vi "CASE.vi"() -> ()   [LabVIEW 2020]
panel:
  out "WARNING":string
  out "Boolean 5":bool
  in  "error out":errorcluster
  out "decimal integer string":string
  in  "Knob":u8(knob) scale=0.0..10.0
  in  "String 2":string
  out "Boolean 4":bool
  out "Boolean 3":bool
  out "Boolean 2":bool
  out "String":string
  in  "Boolean":bool
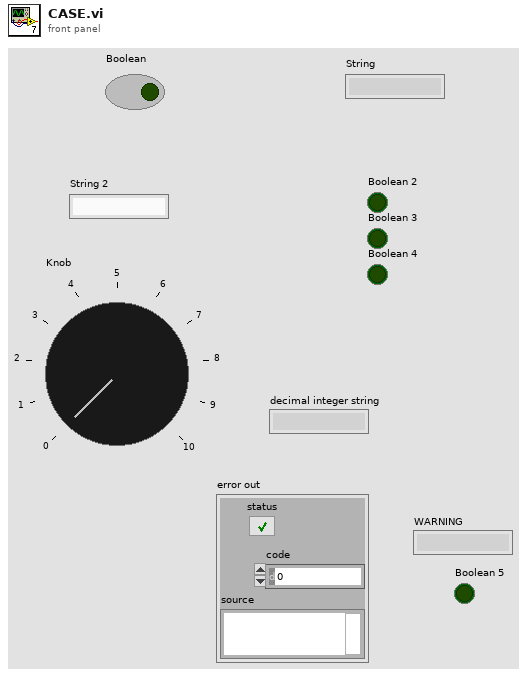
[diagram p1: front panel]
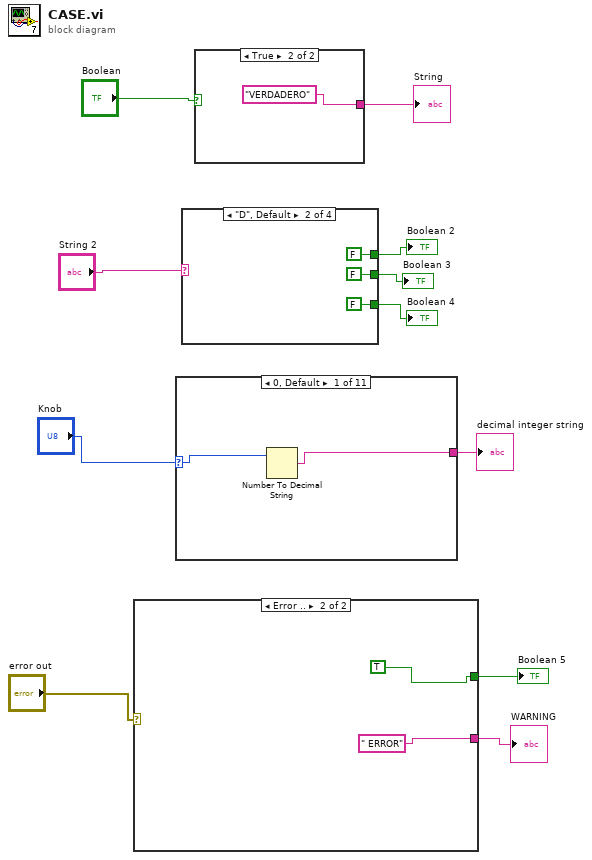
[diagram p0: block diagram]
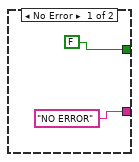
[diagram p2: hidden frame]
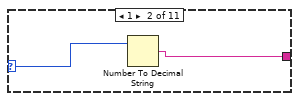
[diagram p3: hidden frame]
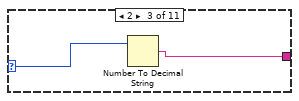
[diagram p4: hidden frame]
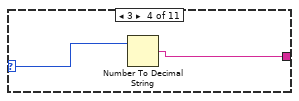
[diagram p5: hidden frame]
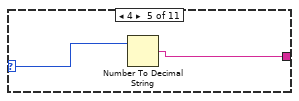
[diagram p6: hidden frame]
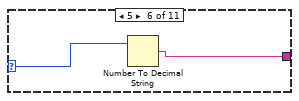
[diagram p7: hidden frame]
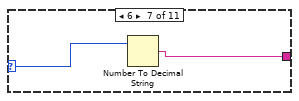
[diagram p8: hidden frame]
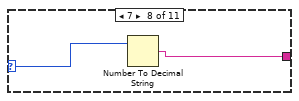
[diagram p9: hidden frame]
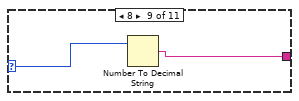
[diagram p10: hidden frame]
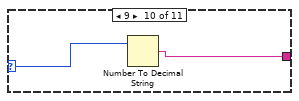
[diagram p11: hidden frame]
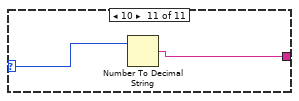
[diagram p12: hidden frame]
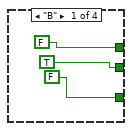
[diagram p13: hidden frame]
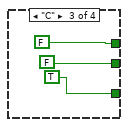
[diagram p14: hidden frame]
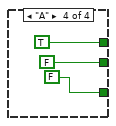
[diagram p15: hidden frame]
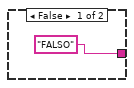
[diagram p16: hidden frame]
diagram:
  n1 = case shown="Error .." "error out" {
    tunnel: [FALSE TRUE] -> w2
    tunnel: ["NO ERROR" ("String") " ERROR" ("String")] -> w1
    frame No Error {
    }
    frame Error {
    }
  }
  "Boolean 5" <- w2
  "WARNING" <- w1
  n2 = case shown="0, Default" "Knob" {
    selector: "Knob" -> [w17 w19 w21 w23 w25 w27 w29 w31 w33 w35 w37]
    tunnel: [w16 w18 w20 w22 w24 w26 w28 w30 w32 w34 w36] -> w4
    frame 0, Default {
      n3 = Number To Decimal String(number=w17) -> (decimal integer string=w16:string)  [unwired: 1 in]
    }
    frame 1 {
      n4 = Number To Decimal String(number=w19) -> (decimal integer string=w18:string)  [unwired: 1 in]
    }
    frame 2 {
      n5 = Number To Decimal String(number=w21) -> (decimal integer string=w20:string)  [unwired: 1 in]
    }
    frame 3 {
      n6 = Number To Decimal String(number=w23) -> (decimal integer string=w22:string)  [unwired: 1 in]
    }
    frame 4 {
      n7 = Number To Decimal String(number=w25) -> (decimal integer string=w24:string)  [unwired: 1 in]
    }
    frame 5 {
      n8 = Number To Decimal String(number=w27) -> (decimal integer string=w26:string)  [unwired: 1 in]
    }
    frame 6 {
      n9 = Number To Decimal String(number=w29) -> (decimal integer string=w28:string)  [unwired: 1 in]
    }
    frame 7 {
      n10 = Number To Decimal String(number=w31) -> (decimal integer string=w30:string)  [unwired: 1 in]
    }
    frame 8 {
      n11 = Number To Decimal String(number=w33) -> (decimal integer string=w32:string)  [unwired: 1 in]
    }
    frame 9 {
      n12 = Number To Decimal String(number=w35) -> (decimal integer string=w34:string)  [unwired: 1 in]
    }
    frame 10 {
      n13 = Number To Decimal String(number=w37) -> (decimal integer string=w36:string)  [unwired: 1 in]
    }
  }
  "decimal integer string" <- w4
  n14 = case shown="\"D\", Default" "String 2" {
    tunnel: [FALSE FALSE FALSE TRUE] -> w8
    tunnel: [TRUE FALSE FALSE FALSE] -> w7
    tunnel: [FALSE FALSE TRUE FALSE] -> w6
    frame "B" {
    }
    frame "D", Default {
    }
    frame "C" {
    }
    frame "A" {
    }
  }
  "Boolean 2" <- w8
  "Boolean 3" <- w7
  "Boolean 4" <- w6
  n15 = case shown="True" "Boolean" {
    tunnel: ["FALSO" ("String") "VERDADERO" ("String")] -> w10
    frame False {
    }
    frame True {
    }
  }
  "String" <- w10
